vi "Conversion_API_Hierarchy.vi"   [LabVIEW 2021]
uses:
  Abs_Types/String/Abs_String.lvclass
  Abs_Types/Single Float/Abs_Single Float.lvclass
  Abs_Types/Double Float/Abs_Double Float.lvclass
  Abs_Types/Extended Float/Abs_Extended Float.lvclass
  Abs_Types/Complex Single Float/Abs_Complex Single Float.lvclass
  Abs_Types/Complex Double Float/Abs_Complex Double Float.lvclass
  Abs_Types/Complex Extended Float/Abs_Complex Extended Float.lvclass
  Abs_Types/I8 Integer/Abs_I8 Integer.lvclass
  Abs_Types/I16 Integer/Abs_I16 Integer.lvclass
  Abs_Types/I32 Integer/Abs_I32 Integer.lvclass
  Abs_Types/I64 Integer/Abs_I64 Integer.lvclass
  Abs_Types/U8 Integer/Abs_U8 Integer.lvclass
  Abs_Types/U16 Integer/Abs_U16 Integer.lvclass
  Abs_Types/U32 Integer/Abs_U32 Integer.lvclass
  Abs_Types/U64 Integer/Abs_U64 Integer.lvclass
  Support/SGL/ConvertTo_SGL.lvclass
  Support/String/ConvertTo_String.lvclass
  Support/JSON/ConvertTo_JSON.lvclass
  Support/Binary/ConvertTo_Binary.lvclass
  Support/DBL/ConvertTo_DBL.lvclass
  Support/EXT/ConvertTo_EXT.lvclass
  Support/CPLX_SGL/ConvertTo_CPLX_SGL.lvclass
  Support/CPLX_DBL/ConvertTo_CPLX_DBL.lvclass
  Support/CPLX_EXT/ConvertTo_CPLX_EXT.lvclass
  Support/I8/ConvertTo_I8.lvclass
  Support/I16/ConvertTo_I16.lvclass
  Support/I32/ConvertTo_I32.lvclass
  Support/I64/ConvertTo_I64.lvclass
  Support/U8/ConvertTo_U8.lvclass
  Support/U16/ConvertTo_U16.lvclass
  Support/U32/ConvertTo_U32.lvclass
  Support/U64/ConvertTo_U64.lvclass
panel:
  # "SEE DIAGRAM\nFOR Hierarchy"
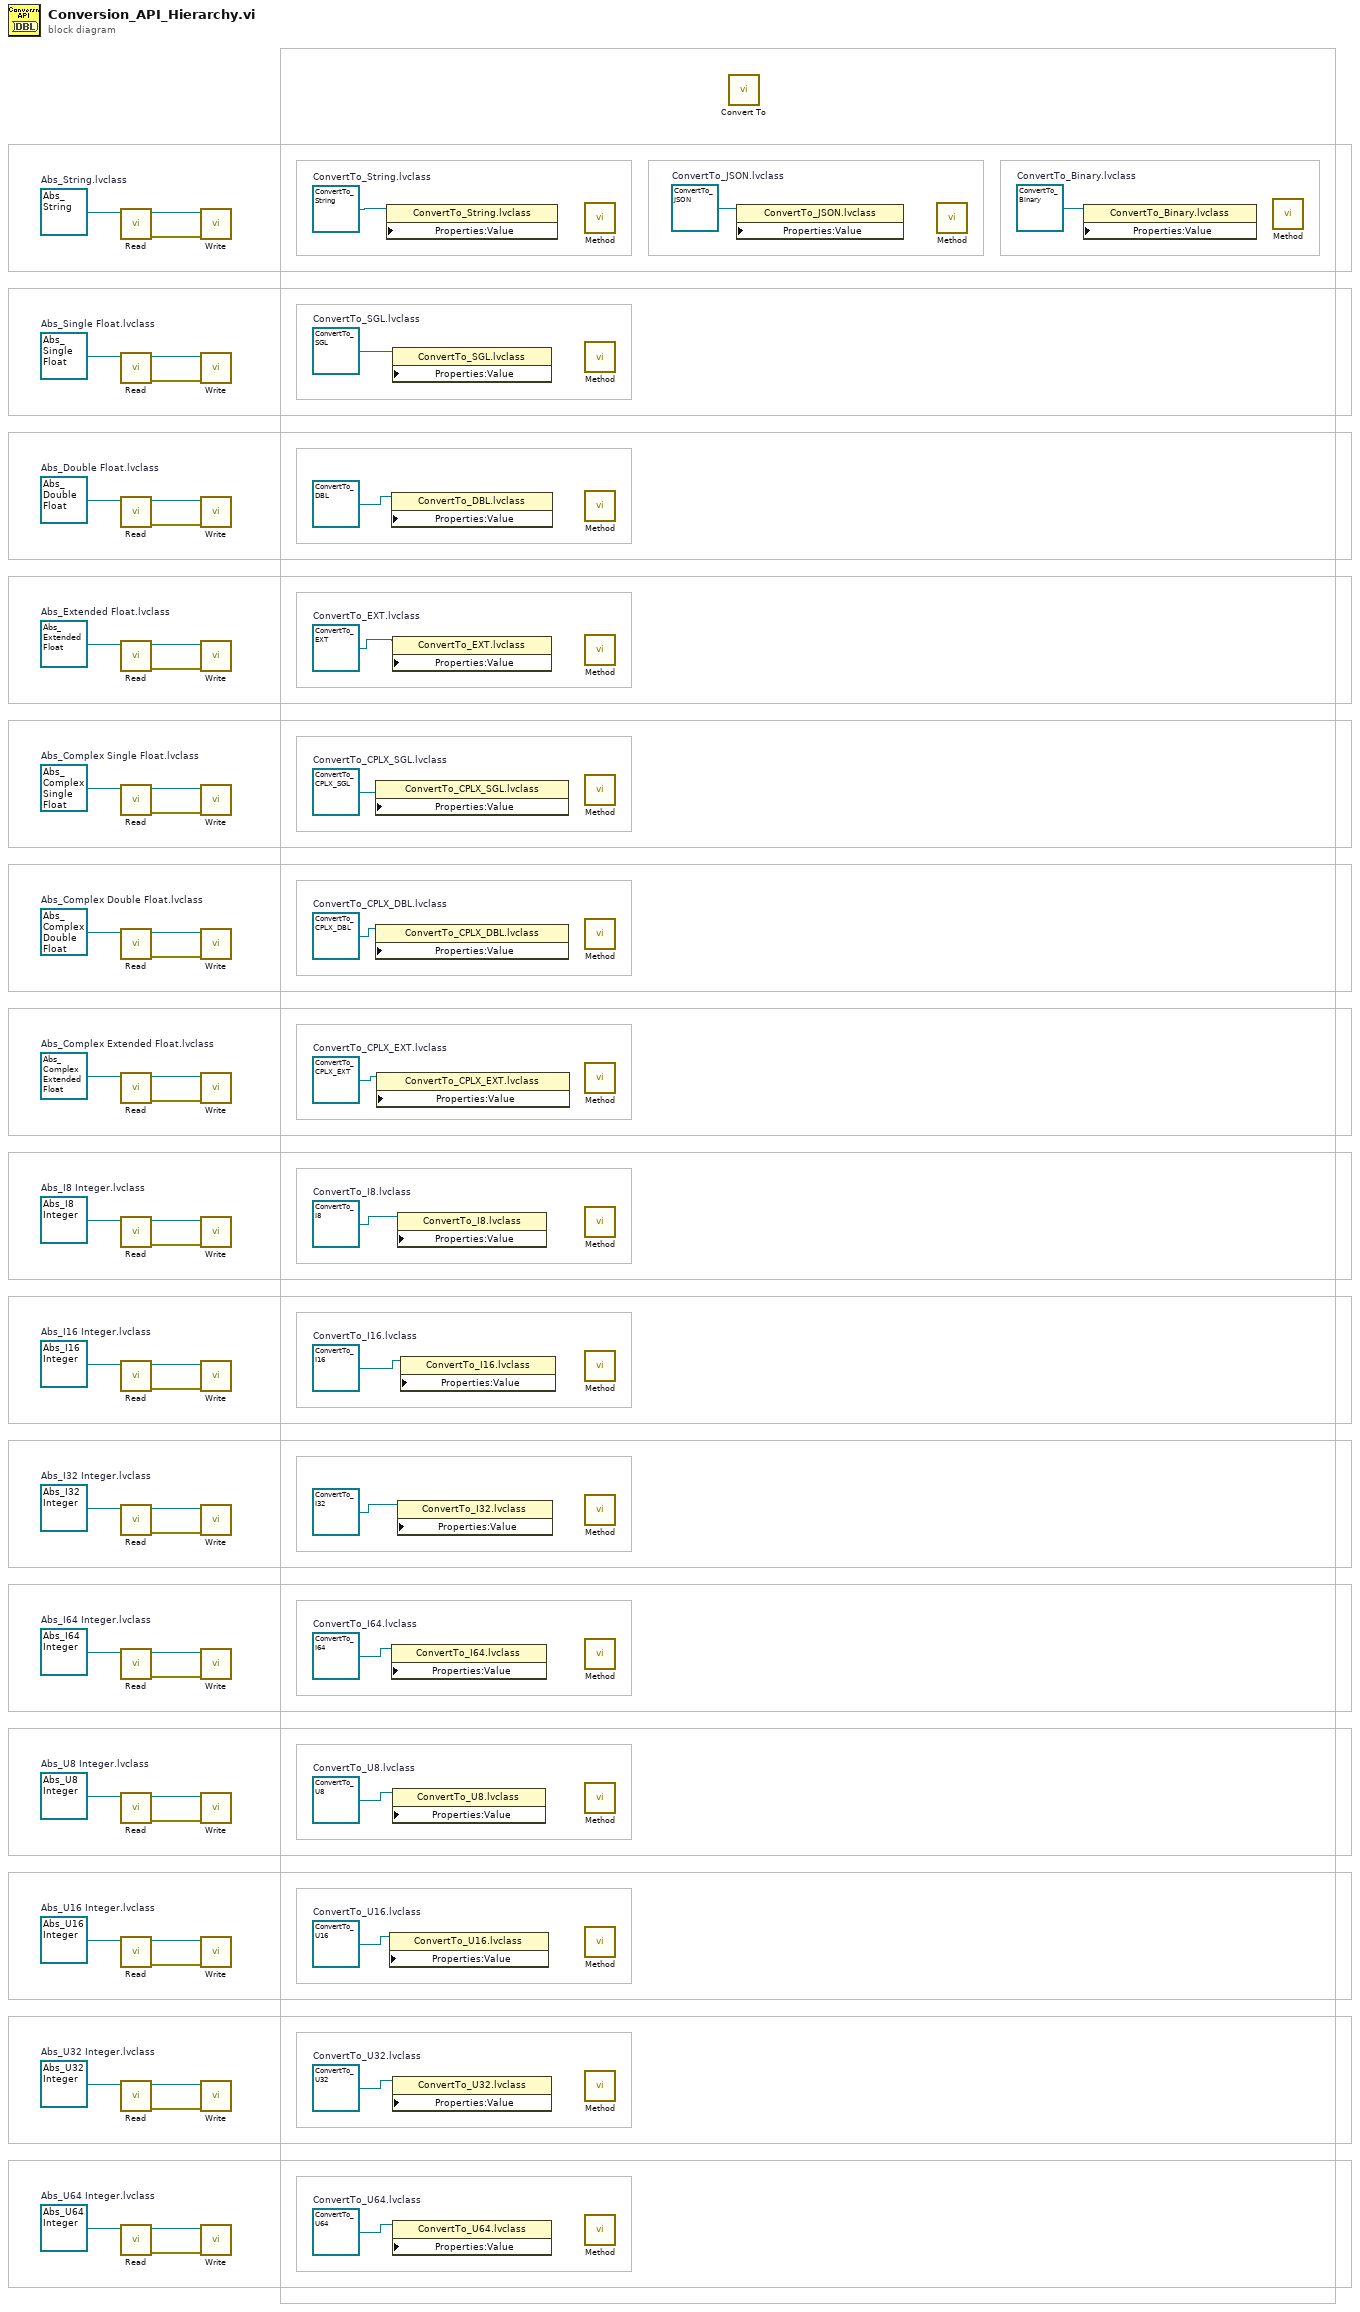
[diagram p0: block diagram]
diagram:
  w3 = refnum<class "ConvertTo_U64.lvclass"> refnum  # ConvertTo_U64.lvclass
  w4 = refnum<class "ConvertTo_U32.lvclass"> refnum  # ConvertTo_U32.lvclass
  w5 = refnum<class "ConvertTo_U16.lvclass"> refnum  # ConvertTo_U16.lvclass
  w6 = refnum<class "ConvertTo_U8.lvclass"> refnum  # ConvertTo_U8.lvclass
  w7 = refnum<class "ConvertTo_I64.lvclass"> refnum  # ConvertTo_I64.lvclass
  w9 = refnum<class "ConvertTo_I16.lvclass"> refnum  # ConvertTo_I16.lvclass
  w10 = refnum<class "ConvertTo_I8.lvclass"> refnum  # ConvertTo_I8.lvclass
  w11 = refnum<class "ConvertTo_CPLX_EXT.lvclass"> refnum  # ConvertTo_CPLX_EXT.lvclass
  w12 = refnum<class "ConvertTo_CPLX_DBL.lvclass"> refnum  # ConvertTo_CPLX_DBL.lvclass
  w13 = refnum<class "ConvertTo_CPLX_SGL.lvclass"> refnum  # ConvertTo_CPLX_SGL.lvclass
  w2 = refnum<class "ConvertTo_EXT.lvclass"> refnum  # ConvertTo_EXT.lvclass
  w14 = refnum<class "ConvertTo_Binary.lvclass"> refnum  # ConvertTo_Binary.lvclass
  w15 = refnum<class "ConvertTo_JSON.lvclass"> refnum  # ConvertTo_JSON.lvclass
  w16 = refnum<class "ConvertTo_String.lvclass"> refnum  # ConvertTo_String.lvclass
  w17 = refnum<class "ConvertTo_SGL.lvclass"> refnum  # ConvertTo_SGL.lvclass
  w20 = refnum<class "Abs_U64 Integer.lvclass"> refnum  # Abs_U64 Integer.lvclass
  w23 = refnum<class "Abs_U32 Integer.lvclass"> refnum  # Abs_U32 Integer.lvclass
  w26 = refnum<class "Abs_U16 Integer.lvclass"> refnum  # Abs_U16 Integer.lvclass
  w29 = refnum<class "Abs_U8 Integer.lvclass"> refnum  # Abs_U8 Integer.lvclass
  w30 = refnum<class "Abs_I64 Integer.lvclass"> refnum  # Abs_I64 Integer.lvclass
  w35 = refnum<class "Abs_I32 Integer.lvclass"> refnum  # Abs_I32 Integer.lvclass
  w38 = refnum<class "Abs_I16 Integer.lvclass"> refnum  # Abs_I16 Integer.lvclass
  w41 = refnum<class "Abs_I8 Integer.lvclass"> refnum  # Abs_I8 Integer.lvclass
  w44 = refnum<class "Abs_Complex Extended Float.lvclass"> refnum  # Abs_Complex Extended Float.lvclass
  w47 = refnum<class "Abs_Complex Double Float.lvclass"> refnum  # Abs_Complex Double Float.lvclass
  w50 = refnum<class "Abs_Complex Single Float.lvclass"> refnum  # Abs_Complex Single Float.lvclass
  w53 = refnum<class "Abs_Extended Float.lvclass"> refnum  # Abs_Extended Float.lvclass
  w56 = refnum<class "Abs_Double Float.lvclass"> refnum  # Abs_Double Float.lvclass
  w59 = refnum<class "Abs_Single Float.lvclass"> refnum  # Abs_Single Float.lvclass
  w60 = refnum<class "Abs_String.lvclass"> refnum  # Abs_String.lvclass
  n1 = call-dynamic "Read.vi"("Abs_String in"=w60) -> ("error out"=w62:errorcluster, "Abs_String out"=w61:refnum<class "Abs_String.lvclass">)  [unwired: 8 in, 1 out]
  n2 = call-dynamic "Read.vi"("Double Float.lvclass_340760 in"=w59) -> ("error out"=w57:errorcluster, "Double Float.lvclass_340760 out"=w58:refnum<class "Abs_Single Float.lvclass">)  [unwired: 8 in, 1 out]
  n3 = call-dynamic "Read.vi"("Double Float.lvclass_340760 in"=w56) -> ("error out"=w54:errorcluster, "Double Float.lvclass_340760 out"=w55:refnum<class "Abs_Double Float.lvclass">)  [unwired: 8 in, 1 out]
  n4 = call-dynamic "Read.vi"("Double Float.lvclass_340760 in"=w53) -> ("error out"=w51:errorcluster, "Double Float.lvclass_340760 out"=w52:refnum<class "Abs_Extended Float.lvclass">)  [unwired: 8 in, 1 out]
  n5 = call-dynamic "Read.vi"("Double Float.lvclass_340760 in"=w50) -> ("error out"=w48:errorcluster, "Double Float.lvclass_340760 out"=w49:refnum<class "Abs_Complex Single Float.lvclass">)  [unwired: 8 in, 1 out]
  n6 = call-dynamic "Read.vi"("Double Float.lvclass_340760 in"=w47) -> ("error out"=w45:errorcluster, "Double Float.lvclass_340760 out"=w46:refnum<class "Abs_Complex Double Float.lvclass">)  [unwired: 8 in, 1 out]
  n7 = call-dynamic "Read.vi"("Double Float.lvclass_340760 in"=w44) -> ("error out"=w42:errorcluster, "Double Float.lvclass_340760 out"=w43:refnum<class "Abs_Complex Extended Float.lvclass">)  [unwired: 8 in, 1 out]
  n8 = call-dynamic "Read.vi"("Double Float.lvclass_340760 in"=w41) -> ("error out"=w39:errorcluster, "Double Float.lvclass_340760 out"=w40:refnum<class "Abs_I8 Integer.lvclass">)  [unwired: 8 in, 1 out]
  n9 = call-dynamic "Read.vi"("Double Float.lvclass_340760 in"=w38) -> ("error out"=w36:errorcluster, "Double Float.lvclass_340760 out"=w37:refnum<class "Abs_I16 Integer.lvclass">)  [unwired: 8 in, 1 out]
  n10 = call-dynamic "Read.vi"("Double Float.lvclass_340760 in"=w35) -> ("error out"=w33:errorcluster, "Double Float.lvclass_340760 out"=w34:refnum<class "Abs_I32 Integer.lvclass">)  [unwired: 8 in, 1 out]
  n11 = call-dynamic "Read.vi"("Double Float.lvclass_340760 in"=w30) -> ("error out"=w31:errorcluster, "Double Float.lvclass_340760 out"=w32:refnum<class "Abs_I64 Integer.lvclass">)  [unwired: 8 in, 1 out]
  n12 = call-dynamic "Read.vi"("Double Float.lvclass_340760 in"=w29) -> ("error out"=w27:errorcluster, "Double Float.lvclass_340760 out"=w28:refnum<class "Abs_U8 Integer.lvclass">)  [unwired: 8 in, 1 out]
  n13 = call-dynamic "Read.vi"("Double Float.lvclass_340760 in"=w26) -> ("error out"=w24:errorcluster, "Double Float.lvclass_340760 out"=w25:refnum<class "Abs_U16 Integer.lvclass">)  [unwired: 8 in, 1 out]
  n14 = call-dynamic "Read.vi"("Double Float.lvclass_340760 in"=w23) -> ("error out"=w21:errorcluster, "Double Float.lvclass_340760 out"=w22:refnum<class "Abs_U32 Integer.lvclass">)  [unwired: 8 in, 1 out]
  n15 = call-dynamic "Read.vi"("Double Float.lvclass_340760 in"=w20) -> ("error out"=w18:errorcluster, "Double Float.lvclass_340760 out"=w19:refnum<class "Abs_U64 Integer.lvclass">)  [unwired: 8 in, 1 out]
  n16 = call-dynamic "Write.vi"("error in (no error)"=w62, "Abs_String in"=w61) -> ()  [unwired: 8 in, 2 out]
  n17 = call-dynamic "Write.vi"("error in (no error)"=w57, "Double Float.lvclass_340760 in"=w58) -> ()  [unwired: 8 in, 2 out]
  n18 = call-dynamic "Write.vi"("error in (no error)"=w54, "Double Float.lvclass in"=w55) -> ()  [unwired: 8 in, 2 out]
  n19 = call-dynamic "Write.vi"("error in (no error)"=w51, "Double Float.lvclass_340760 in"=w52) -> ()  [unwired: 8 in, 2 out]
  n20 = call-dynamic "Write.vi"("error in (no error)"=w48, "Double Float.lvclass_340760 in"=w49) -> ()  [unwired: 8 in, 2 out]
  n21 = call-dynamic "Write.vi"("error in (no error)"=w45, "Double Float.lvclass_340760 in"=w46) -> ()  [unwired: 8 in, 2 out]
  n22 = call-dynamic "Write.vi"("error in (no error)"=w42, "Double Float.lvclass_340760 in"=w43) -> ()  [unwired: 8 in, 2 out]
  n23 = call-dynamic "Write.vi"("error in (no error)"=w39, "Double Float.lvclass_340760 in"=w40) -> ()  [unwired: 8 in, 2 out]
  n24 = call-dynamic "Write.vi"("error in (no error)"=w36, "Double Float.lvclass_340760 in"=w37) -> ()  [unwired: 8 in, 2 out]
  n25 = call-dynamic "Write.vi"("error in (no error)"=w33, "Double Float.lvclass_340760 in"=w34) -> ()  [unwired: 8 in, 2 out]
  n26 = call-dynamic "Write.vi"("error in (no error)"=w31, "Double Float.lvclass_340760 in"=w32) -> ()  [unwired: 8 in, 2 out]
  n27 = call-dynamic "Write.vi"("error in (no error)"=w27, "Double Float.lvclass_340760 in"=w28) -> ()  [unwired: 8 in, 2 out]
  n28 = call-dynamic "Write.vi"("error in (no error)"=w24, "Double Float.lvclass_340760 in"=w25) -> ()  [unwired: 8 in, 2 out]
  n29 = call-dynamic "Write.vi"("error in (no error)"=w21, "Double Float.lvclass_340760 in"=w22) -> ()  [unwired: 8 in, 2 out]
  n30 = call-dynamic "Write.vi"("error in (no error)"=w18, "Double Float.lvclass_340760 in"=w19) -> ()  [unwired: 8 in, 2 out]
  n31 = property class="ConvertTo_CPLX_SGL.lvclass" props=["Properties:Value"](reference=w13) -> ()  [unwired: 2 in, 2 out]
  n32 = property class="ConvertTo_CPLX_DBL.lvclass" props=["Properties:Value"](reference=w12) -> ()  [unwired: 2 in, 2 out]
  n33 = property class="ConvertTo_CPLX_EXT.lvclass" props=["Properties:Value"](reference=w11) -> ()  [unwired: 2 in, 2 out]
  n34 = property class="ConvertTo_String.lvclass" props=["Properties:Value"](reference=w16) -> ()  [unwired: 2 in, 2 out]
  n35 = property class="ConvertTo_U16.lvclass" props=["Properties:Value"](reference=w5) -> ()  [unwired: 2 in, 2 out]
  n36 = property class="ConvertTo_DBL.lvclass" props=["Properties:Value"](reference=refnum<class "ConvertTo_DBL.lvclass"> refnum ("ConvertTo_DBL.lvclass")) -> ()  [unwired: 2 in, 2 out]
  n37 = property class="ConvertTo_I64.lvclass" props=["Properties:Value"](reference=w7) -> ()  [unwired: 2 in, 2 out]
  n38 = property class="ConvertTo_SGL.lvclass" props=["Properties:Value"](reference=w17) -> ()  [unwired: 2 in, 2 out]
  n39 = property class="ConvertTo_EXT.lvclass" props=["Properties:Value"](reference=w2) -> ()  [unwired: 2 in, 2 out]
  n40 = property class="ConvertTo_U8.lvclass" props=["Properties:Value"](reference=w6) -> ()  [unwired: 2 in, 2 out]
  n41 = property class="ConvertTo_U32.lvclass" props=["Properties:Value"](reference=w4) -> ()  [unwired: 2 in, 2 out]
  n42 = property class="ConvertTo_U64.lvclass" props=["Properties:Value"](reference=w3) -> ()  [unwired: 2 in, 2 out]
  n43 = property class="ConvertTo_I8.lvclass" props=["Properties:Value"](reference=w10) -> ()  [unwired: 2 in, 2 out]
  n44 = property class="ConvertTo_I32.lvclass" props=["Properties:Value"](reference=refnum<class "ConvertTo_I32.lvclass"> refnum ("ConvertTo_I32.lvclass")) -> ()  [unwired: 2 in, 2 out]
  n45 = property class="ConvertTo_I16.lvclass" props=["Properties:Value"](reference=w9) -> ()  [unwired: 2 in, 2 out]
  n46 = call "Method.vi"() -> ()  [unwired: 5 in, 1 out]
  n47 = call "Method.vi"() -> ()  [unwired: 5 in, 1 out]
  n48 = call "Method.vi"() -> ()  [unwired: 5 in, 1 out]
  n49 = call "Method.vi"() -> ()  [unwired: 5 in, 1 out]
  n50 = call "Method.vi"() -> ()  [unwired: 5 in, 1 out]
  n51 = call "Method.vi"() -> ()  [unwired: 5 in, 1 out]
  n52 = call "Method.vi"() -> ()  [unwired: 5 in, 1 out]
  n53 = call "Method.vi"() -> ()  [unwired: 5 in, 1 out]
  n54 = call "Method.vi"() -> ()  [unwired: 5 in, 1 out]
  n55 = call "Method.vi"() -> ()  [unwired: 5 in, 1 out]
  n56 = call "Method.vi"() -> ()  [unwired: 5 in, 1 out]
  n57 = call "Method.vi"() -> ()  [unwired: 5 in, 1 out]
  n58 = call "Method.vi"() -> ()  [unwired: 5 in, 1 out]
  n59 = call "Method.vi"() -> ()  [unwired: 5 in, 1 out]
  n60 = call "Method.vi"() -> ()  [unwired: 5 in, 1 out]
  n61 = call-poly "Convert To.vi"() -> ()  [unwired: 5 in, 1 out]
  n62 = property class="ConvertTo_JSON.lvclass" props=["Properties:Value"](reference=w15) -> ()  [unwired: 2 in, 2 out]
  n63 = call "Method.vi"() -> ()  [unwired: 5 in, 1 out]
  n64 = property class="ConvertTo_Binary.lvclass" props=["Properties:Value"](reference=w14) -> ()  [unwired: 2 in, 2 out]
  n65 = call "Method.vi"() -> ()  [unwired: 5 in, 1 out]
